vi "Open Server Connection.vi"(8 "error in (no error)":errorcluster, 9 "Port":u16, 10 "address":string, 11 "RemoteControl.ZMQ in":refnum<class "RemoteControl.ZMQ.lvclass">) -> (0 "error out":errorcluster, 3 "RemoteControl.ZMQ out":refnum<class "RemoteControl.ZMQ.lvclass">)   [LabVIEW 2019, in "RemoteControl.ZMQ.lvclass"]
uses:
  RemoteControl.ZMQ.lvclass
  <vilib>/addons/zeromq/socket_type.ctl
  RemoteControl.ZMQ.lvclass/RemoteControl.ZMQ.ctl
  <vilib>/addons/zeromq/zmq_context.lvclass
  <vilib>/addons/zeromq/zmq_socket.lvclass
  <vilib>/addons/zeromq/zeromq.lvlib
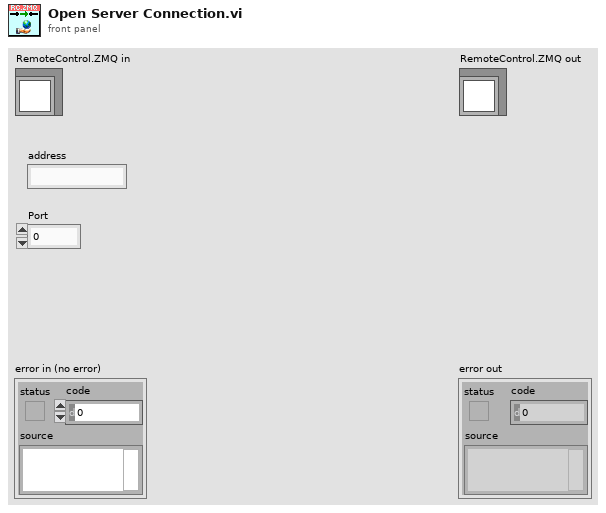
[diagram p1: front panel]
types:
  T1 = typedef "zeromq.lvlib/socket_type.ctl" = enum8{"ZMQ_PAIR", "ZMQ_PUB", "ZMQ_SUB", "ZMQ_REQ", "ZMQ_REP", "ZMQ_DEALER", "ZMQ_ROUTER", "ZMQ_PULL", "ZMQ_PUSH", "ZMQ_XPUB", "ZMQ_XSUB", "ZMQ_STREAM", "ZMQ_SERVER", "ZMQ_CLIENT", "ZMQ_RADIO", "ZMQ_DISH", "ZMQ_GATHER", "ZMQ_SCATTER", "ZMQ_DGRAM"}
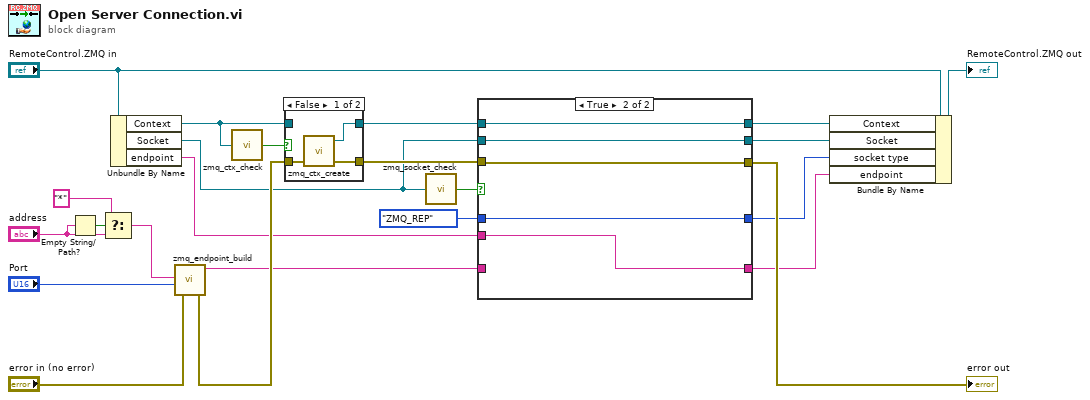
[diagram p0: block diagram]
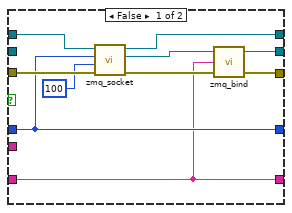
[diagram p3: hidden frame]
diagram:
  n1 = Empty String/Path?(string/path="address") -> (empty?=w19:bool)
  n2 = Select(t="*", s=w19, f="address") -> (s? t:f=w16:string)
  n3 = Unbundle By Name("RemoteControl.ZMQ in") -> ("Context"=w8:refnum<class "zmq_context.lvclass">, "Socket"=w7:refnum<class "zmq_socket.lvclass">, "endpoint"=w3:string)
  n4 = call <vilib>:"zmq_endpoint_build.vi"("error in"="error in (no error)", "port"="Port", "address"=w16) -> ("error out"=w12:errorcluster, "endpoint"=w6:string)  [unwired: 2 in, 1 out]
  n5 = call <vilib>:"zmq_ctx_check.vi"("context in"=w8) -> ("valid?"=w11:bool)
  n6 = case shown="False" w11 {
    tunnel: [w26 w28] -> w14
    tunnel: [w25 w27] -> w13
    tunnel: w12 -> [w24 w27]
    tunnel: w8 -> [_ w28]
    frame False {
      n7 = call <vilib>:"zmq_ctx_create.vi"("error in"=w24) -> ("error out"=w25:errorcluster, "context out"=w26:refnum<class "zmq_context.lvclass">)  [unwired: 3 in]
    }
    frame True {
    }
  }
  n8 = call <vilib>:"zmq_socket_check.vi"("socket in"=w7) -> ("valid?"=w9:bool)
  n9 = case shown="True" w9 {
    tunnel: socket_type."ZMQ_REP" ("socket type") -> [w30 w43]
    tunnel: [w38 w42] -> w15
    tunnel: w14 -> [w35 w42]
    tunnel: w13 -> [w37 w40]
    tunnel: w7 -> [_ w41]
    tunnel: [w30 w43] -> w1
    tunnel: [w31 w41] -> w4
    tunnel: w6 -> [w29 _]
    tunnel: [w32 w40] -> w5
    tunnel: w3 -> [_ w39]
    tunnel: [w29 w39] -> w2
    frame False {
      n10 = call <vilib>:"zmq_socket.vi"("error in"=w37, "linger (ms)"=100, "socket type"=w30, "context in"=w35) -> ("error out"=w34:errorcluster, "socket out"=w33:refnum<class "zmq_socket.lvclass">, "context out"=w38:refnum<class "zmq_context.lvclass">)  [unwired: 1 in]
      n11 = call <vilib>:"zmq_bind.vi"("error in"=w34, "endpoint"=w29, "socket in"=w33) -> ("error out"=w32:errorcluster, "socket out"=w31:refnum<class "zmq_socket.lvclass">)  [unwired: 1 in]
    }
    frame True {
    }
  }
  "error out" <- w5
  n12 = Bundle By Name(cluster="RemoteControl.ZMQ in", "Context"=w15, "Socket"=w4, "socket type"=w1, "endpoint"=w2) -> (→"RemoteControl.ZMQ out":refnum<class "RemoteControl.ZMQ.lvclass">)
